vi "case-counter.vi"(10 "reset":bool) -> (2 "count":i16)   [LabVIEW 2015, in "libimaging-cs.lvlib"]
uses:
  libimaging-cs.lvlib
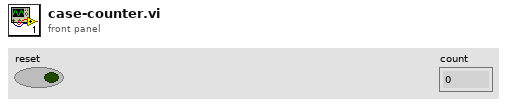
[diagram p1: front panel]
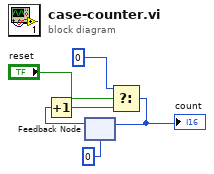
[diagram p0: block diagram]
diagram:
  n1 = feedback #1(i16 0) -> (w2:i16)
  n2 = Increment(x=w2) -> (x+1=w6:i16)
  n3 = Select(t=i16 0, s="reset", f=w6) -> (s? t:f=w3:i16)
  "count" <- w3
  n4 = feedback-in #1(w3) -> ()
